vi "Get Project Item.vi"(6 "project item file extension":string=".lvlib", 7 "error if not found":bool=TRUE, 8 "error in (no error)":errorcluster, 9 "project item type":string="Library", 10 "project item name":string, 11 "project in":refnum<vi>) -> (0 "error out":errorcluster, 1 "found":bool, 2 "project item":refnum<vi>, 3 "project out":refnum<vi>)   [LabVIEW 2021, in "MeasurementService Editor.lvlib"]
uses:
  MeasurementService Editor.lvlib
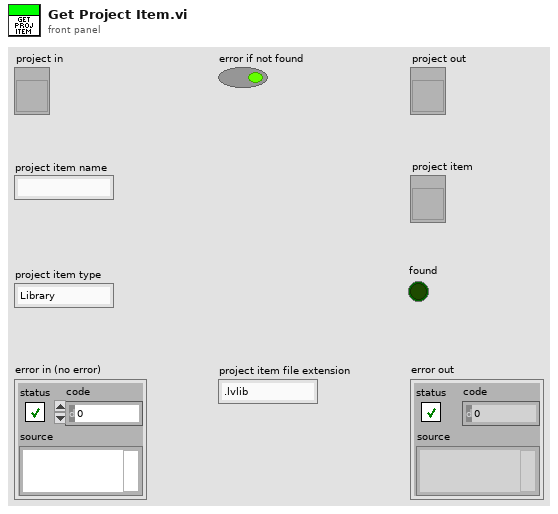
[diagram p1: front panel]
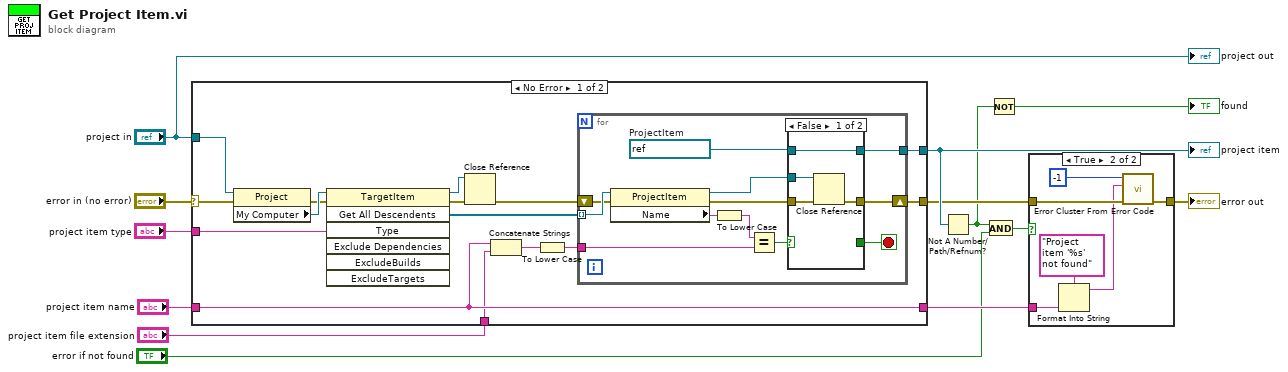
[diagram p0: block diagram]
diagram:
  n1 = case shown="No Error" "error in (no error)" {
    selector: "error in (no error)" -> [w24 w49]
    tunnel: "project in" -> [w28 _]
    tunnel: "project item name" -> [w18 w48]
    tunnel: [w23 w49] -> w8
    tunnel: [w19 _] -> w10
    tunnel: [w18 w48] -> w7
    tunnel: "project item type" -> [w17 _]
    tunnel: "project item file extension" -> [w15 _]
    frame No Error {
      n2 = property class="Project"(reference=w28, error in=w24) -> (error out=w26:errorcluster, "My Computer"=w27:refnum<vi>)  [unwired: 1 out]
      n3 = invoke class="TargetItem" method="Get All Descendents"(reference=w27, error in=w26, "Type"=w17) -> (reference out=w21:refnum<vi>, error out=w22:errorcluster, "All Descendents"=w25:refnum<vi>[])  [unwired: 4 in, 4 out]
      n4 = Close Reference(reference=w21, error in (no error)=w22) -> (error out=w20:errorcluster)
      n5 = Concatenate Strings(w18, w15) -> (w16:string)
      n6 = To Lower Case(string=w16) -> (all lower case string=w14:string)
      n7 = for {
        tunnel: w25 -> [w40] mode=indexing
        shift-right: [w35] -> w23
        shift-left: w20 -> [w39]
        tunnel: [w34] -> w19
        tunnel: w14 -> [w29]
        stop <- w31 stop-if-true
        w30 = refnum<vi> refnum  # ProjectItem
        n8 = property class="ProjectItem"(reference=w40, error in=w39) -> (reference out=w37:refnum<vi>, error out=w38:errorcluster, "Name"=w33:string)
        n9 = To Lower Case(string=w33) -> (all lower case string=w32:string)
        n10 = Equal?(x=w32, y=w29) -> (x = y?=w36:bool)
        n11 = case shown="False" w36 {
          selector: w36 -> [_ w45]
          tunnel: w38 -> [w44 w47]
          tunnel: w37 -> [w41 w46]
          tunnel: [w43 w47] -> w35
          tunnel: [w42 w46] -> w34
          tunnel: w30 -> [w42 _]
          tunnel: [_ w45] -> w31
          frame False {
            n12 = Close Reference(reference=w41, error in (no error)=w44) -> (error out=w43:errorcluster)
          }
          frame True {
          }
        }
      }
    }
    frame Error {
    }
  }
  "project item" <- w10
  n13 = Not A Number/Path/Refnum?(number/path/refnum=w10) -> (NaN/Path/Refnum?=w4:bool)
  n14 = And(x=w4, y="error if not found") -> (x .and. y?=w6:bool)
  n15 = Not(x=w4) -> (.not. x?=→"found":bool)
  n16 = case shown="True" w6 {
    tunnel: [w50 w56] -> w9
    tunnel: w8 -> [w50 w55]
    tunnel: w7 -> [_ w51]
    frame False {
    }
    frame True {
      n17 = Format Into String(format string="Project item '%s' not found" ("initial string"), w51) -> (resulting string=w52:string)  [unwired: 2 in, 1 out]
      n18 = call <vilib>:"Error Cluster From Error Code.vi"("error in (no error)"=w55, "error message (\"\")"=w52, "error code (0)"=-1) -> ("error out"=w56:errorcluster)  [unwired: 6 in]
    }
  }
  "error out" <- w9
  "project out" <- "project in"
